vi "save_data_drive.vi"(10 "element 2":string, 11 "element":string) -> ()   [LabVIEW 2021]
uses:
  <vilib>/Utility/file.llb/Write Delimited Spreadsheet (string).vi
panel:
  out "new file path (Not A Path if cancelled)":path
  out "error out":errorcluster
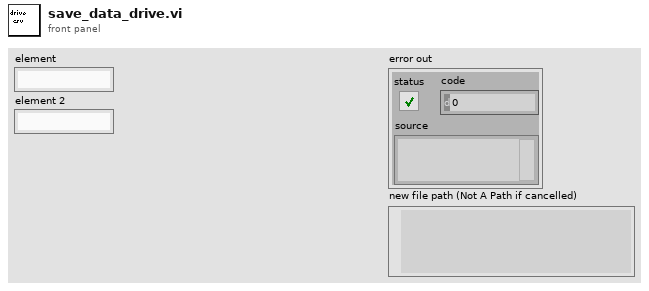
[diagram p1: front panel]
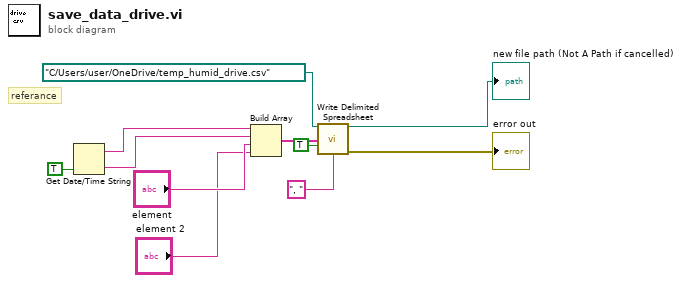
[diagram p0: block diagram]
diagram:
  # "referance"
  n1 = Get Date/Time String(want seconds? (F)=TRUE) -> (date string=w6:string, time string=w5:string)  [unwired: 2 in]
  n2 = Build Array(w6, w5, "element", "element 2") -> (w2:string[])
  n3 = call-poly <vilib>:"Write Delimited Spreadsheet.vi"("file path (dialog if empty)"=path "C:/Users/user/OneDrive/temp_humid_drive.csv", "1D data"=w2, "append to file? (new file:F)"=TRUE, "delimiter (\\t)"=", " ("delimiter (\\t)")) -> ("new file path (Not A Path if cancelled)"=→"new file path (Not A Path if cancelled)":path, "error out"=→"error out":errorcluster)  [unwired: 10 in]
